vi "Sensor Data (Multiple Readings).vi"(6 "Reading Interval (100)":dbl=100.0, 7 "Sample Count (1)":i32=1, 8 "error in (no error)":errorcluster, 9 "Data Source (0:Kelvin)":u16(ring) items=["Kelvin", "Celsius", "Sensor Units"], 10 "Input (0:A)":u16(ring) items=["A", "B"], 11 "VISA resource name":refnum<visa-resource-name>) -> (0 "error out":errorcluster, 2 "Sensor Data":dbl[](array[numeric]) format="%.4f", 3 "VISA resource name out":refnum<visa-resource-name>)   [LabVIEW 2019, in "Lake Shore 335.lvlib"]
doc: "Reads and returns multiple sensor readings from the instrument. Control over interval between readings is also provided."
uses:
  Lake Shore 335.lvlib
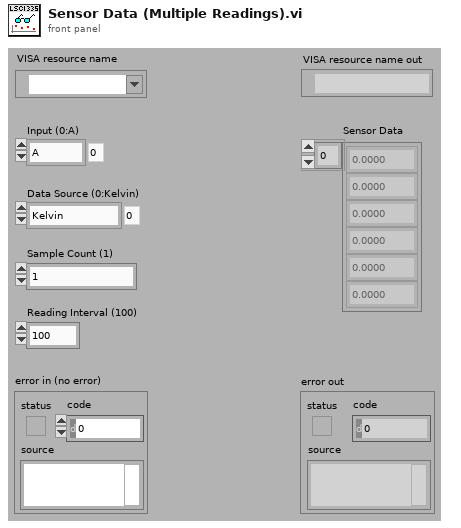
[diagram p1: front panel]
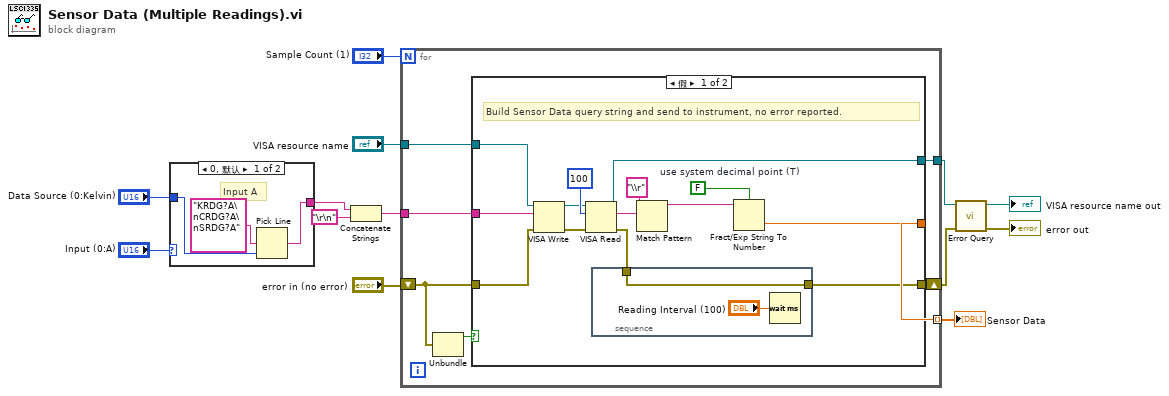
[diagram p0: block diagram]
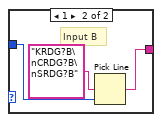
[diagram p2: hidden frame]
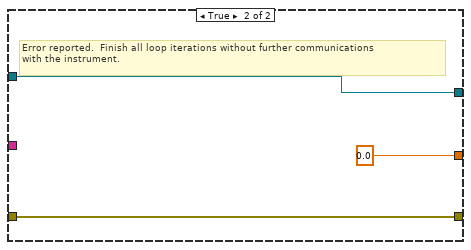
[diagram p3: hidden frame]
diagram:
  n1 = case shown="0, 默认" "Input (0:A)" {
    tunnel: "Data Source (0:Kelvin)" -> [w15 w17]
    tunnel: [w14 w18] -> w4
    frame 0, Default {
      # "Input A"
      n2 = Pick Line(multi-line string="KRDG?A\nCRDG?A\nSRDG?A", line index=w15) -> (output string=w14:string)  [unwired: 1 in]
    }
    frame 1 {
      # "Input B"
      n3 = Pick Line(multi-line string="KRDG?B\nCRDG?B\nSRDG?B", line index=w17) -> (output string=w18:string)  [unwired: 1 in]
    }
  }
  n4 = Concatenate Strings(w4, "\r\n") -> (w3:string)
  n5 = for {
    N: "Sample Count (1)" -> [_]
    tunnel: "VISA resource name" -> [w26]
    tunnel: [w25] -> w10
    tunnel: w3 -> [w24]
    tunnel: [w23] -> w8 mode=indexing
    shift-right: [w22] -> w6
    shift-left: "error in (no error)" -> [w21]
    n6 = Unbundle(w21) -> ("status"=w20:bool)  [unwired: 2 out]
    n7 = case shown="假" w20 {
      tunnel: w26 -> [w40 w45]
      tunnel: [w39 w45] -> w25
      tunnel: w24 -> [w31 _]
      tunnel: [w30 0.0] -> w23
      tunnel: w21 -> [w29 w44]
      tunnel: [w27 w44] -> w22
      frame False {
        w33 = FALSE  # use system decimal point (T)
        # "Build Sensor Data query string and send to instrument, no error reported."
        n8 = VISA Write(VISA resource name=w40, write buffer=w31, error in (no error)=w29) -> (VISA resource name out=w35:refnum<visa-resource-name>, error out=w34:errorcluster)  [unwired: 1 out]
        n9 = VISA Read(VISA resource name=w35, byte count=100, error in (no error)=w34) -> (VISA resource name out=w39:refnum<visa-resource-name>, read buffer=w37:string, error out=w28:errorcluster)  [unwired: 1 out]
        n10 = stacked-sequence {
          tunnel: w28 -> [w41]
          tunnel: [w41] -> w27
          frame #0 {
            n11 = Wait (ms)(milliseconds to wait="Reading Interval (100)") -> ()  [unwired: 1 out]
          }
        }
        n12 = Match Pattern(string=w37, regular expression="\\r") -> (before substring=w32:string)  [unwired: 1 in, 3 out]
        n13 = Fract/Exp String To Number(use system decimal point (T)=w33, string=w32) -> (number=w30:dbl)  [unwired: 2 in, 1 out]
      }
      frame True {
        # "Error reported.  Finish all loop iterations without further communications\nwith the instrument."
      }
    }
  }
  "Sensor Data" <- w8
  n14 = call "Error Query.vi"("error in (no error)"=w6, "VISA resource name"=w10) -> ("error out"=→"error out":errorcluster, "VISA resource name out"=→"VISA resource name out":refnum<visa-resource-name>)  [unwired: 7 in, 1 out]
